vi "DigitalTriggeredAudioNoise.vi"() -> ()   [LabVIEW 2010]
uses:
  <vilib>/DAQmx/read.llb/DAQmx Read (Digital 1D Bool NChan 1Samp 1Line).vi
  <vilib>/DAQmx/create/channels.llb/DAQmx Create Channel (DI-Digital Input).vi
  <vilib>/sound2/lvsound2.llb/Sound Output Write (DBL Single).vi
  <vilib>/daqmx/miscellaneous.llb/DAQmx Fill In Error Info.vi
  <vilib>/measure/NI_MAPro.lvlib
panel:
  out "start frequency":dbl
  out "triggered":bool
  in  "duration (sec)":dbl=2.0
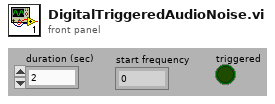
[diagram p1: front panel]
types:
  T1 = typedef "Sound Output Task ID.ctl" = u32
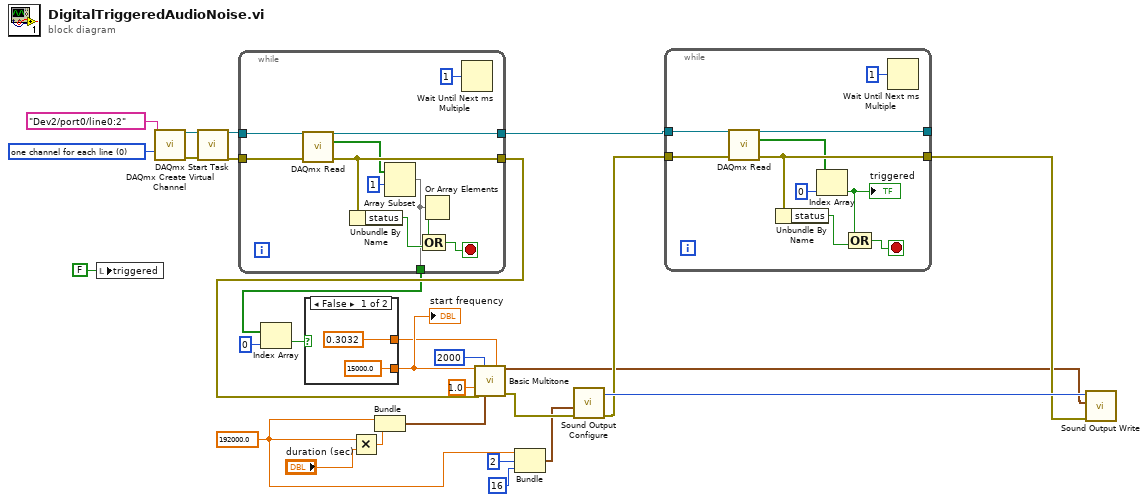
[diagram p0: block diagram]
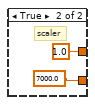
[diagram p2: hidden frame]
diagram:
  w6 = 192000.0 ("x")
  w27 = 0 items=["one channel for each line", "one channel for all lines"] ("line grouping")
  n1 = local write "triggered"(FALSE ("triggered")) -> ()
  n2 = call-poly <vilib>:"DAQmx Create Virtual Channel.vi"("lines"=tag "Dev2/port0/line0:2", "line grouping"=w27) -> ("task out"=w23:refnum<k21>, "error out"=w22:errorcluster)  [unwired: 12 in]
  n3 = call <vilib>:"DAQmx Start Task.vi"("task/channels in"=w23, "error in"=w22) -> ("task out"=w21:refnum<k21>, "error out"=w20:errorcluster)  [unwired: 12 in]
  n4 = while {
    tunnel: w20 -> [w39]
    tunnel: [w36] -> w16
    tunnel: w21 -> [w35]
    tunnel: [w34] -> w19
    tunnel: [w29] -> w13
    stop <- w38 stop-if-true
    n5 = call-poly <vilib>:"DAQmx Read.vi"("task/channels in"=w35, "error in"=w39) -> ("task out"=w34:refnum<k21>, "data"=w30:bool[], "error out"=w36:errorcluster)  [unwired: 11 in]
    n6 = Unbundle By Name(w36) -> ("status"=w37:bool)
    n7 = Array Subset(array=w30, index=1) -> (w29:bool[])  [unwired: 1 in]
    n8 = Or Array Elements(Boolean array=w29) -> (logical OR=w32:bool)
    n9 = Compound Arithmetic op=OR(w32, w37) -> (w38:bool)
    n10 = Wait Until Next ms Multiple(millisecond multiple=u32 1 ("milliseconds to wait")) -> ()  [unwired: 1 out]
  }
  n11 = Index Array(array=w13, index=0) -> (element=w11:bool)
  n12 = case shown="False" w11 {
    tunnel: [15000.0 ("start frequency") 7000.0 ("start frequency")] -> w10
    tunnel: [0.3032 ("amplitude") 1.0 ("amplitude")] -> w2
    frame False {
    }
    frame True {
      # "scaler"
    }
  }
  "start frequency" <- w10
  n13 = Multiply(x=w6, y="duration (sec)") -> (x*y=w7:dbl)
  n14 = Bundle("x"=w6, w7) -> (w8:cluster{"x":dbl, dbl})  [unwired: 1 in]
  n15 = call <vilib>:"Basic Multitone.vi"("start frequency"=w10, "#tones"=2000, "amplitude"=w2, "delta frequency"=1.0, "error in (no error)"=w16, "sampling info"=w8) -> ("signal out"=w14:waveform(dbl), "error out"=w15:errorcluster)  [unwired: 6 in, 2 out]
  n16 = Bundle("x"=w6, 2, 16) -> (w3:cluster{"x":dbl, i32, i32})  [unwired: 1 in]
  n17 = call <vilib>:"Sound Output Configure.vi"("error in (no error)"=w15, "sound format"=w3) -> ("error out"=w25:errorcluster, "task ID"=w28:T1)  [unwired: 8 in]
  n18 = while {
    tunnel: w25 -> [w53]
    tunnel: [w50] -> w24
    tunnel: w19 -> [w49]
    tunnel: [w48] -> _
    stop <- w52 stop-if-true
    n19 = call-poly <vilib>:"DAQmx Read.vi"("task/channels in"=w49, "error in"=w53) -> ("task out"=w48:refnum<k21>, "data"=w46:bool[], "error out"=w50:errorcluster)  [unwired: 11 in]
    n20 = Unbundle By Name(w50) -> ("status"=w51:bool)
    n21 = Index Array(array=w46, index=0) -> (element=w45:bool)
    "triggered" <- w45
    n22 = Compound Arithmetic op=OR(w45, w51) -> (w52:bool)
    n23 = Wait Until Next ms Multiple(millisecond multiple=u32 1 ("milliseconds to wait")) -> ()  [unwired: 1 out]
  }
  n24 = call-poly <vilib>:"Sound Output Write.vi"("error in (no error)"=w24, "data"=w14, "task ID"=w28) -> ()  [unwired: 7 in, 2 out]
